vi "SwerveModuleOdometry.vi"(2 "Module Fault":bool, 3 "Wheel Distance (in)":dbl, 4 "Wheel Azimuth (deg)":dbl, 5 "Robot Heading(deg)":dbl) -> (0 "Delta Y (in)":dbl, 1 "Delta X (in)":dbl)   [LabVIEW 2019]
doc: "This VI calculates the odometry for a single swerve module."
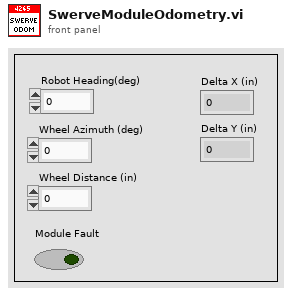
[diagram p1: front panel]
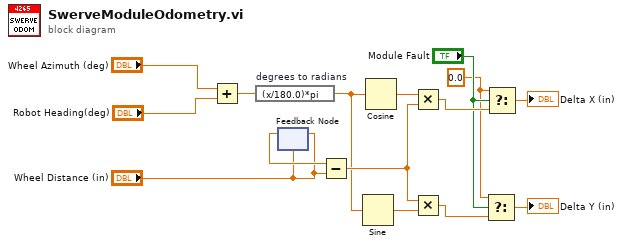
[diagram p0: block diagram]
diagram:
  w2 = 0.0 ("t")
  n1 = Add(x="Wheel Azimuth (deg)", y="Robot Heading(deg)") -> (x+y=w9:dbl)
  n2 = expression code="(x/180.0)*pi" "degrees to radians"(w9) -> (w8:dbl)
  n3 = feedback #1("Wheel Distance (in)") -> (w11:dbl)
  n4 = feedback-in #1("Wheel Distance (in)") -> ()
  n5 = Subtract(x=w11, y="Wheel Distance (in)") -> (x-y=w12:dbl)
  n6 = Sine(x=w8) -> (sin(x)=w13:dbl)
  n7 = Cosine(x=w8) -> (cos(x)=w10:dbl)
  n8 = Multiply(x=w10, y=w12) -> (x*y=w5:dbl)
  n9 = Multiply(x=w12, y=w13) -> (x*y=w4:dbl)
  n10 = Select(t=w2, s="Module Fault", f=w4) -> (s? t:f=→"Delta Y (in)":dbl)
  n11 = Select(t=w2, s="Module Fault", f=w5) -> (s? t:f=→"Delta X (in)":dbl)
